vi "VMS_6_Master.vi"   [LabVIEW 2018]
uses:
  Common_FPGA_Timestamp/DataTypes/TimestampSettings.ctl
  <vilib>/rvi/Emulation/niFpgaGetClockAttributes.vi
  <vilib>/rvi/Emulation/niFpgaSctlEmulationGetInTimedLoop.vi
  <vilib>/rvi/Emulation/niFpgaEmulationReportErrorSimple.vi
  <vilib>/rvi/Emulation/niFpgaEmulationIsFPGAContextNoSignature.vi
  <vilib>/rvi/errors/niFpgaSetErrorForExecOnDevCompSimple.vi
  <vilib>/rvi/eio/common/nirviEmuReportErrorAndStop.vi
  <vilib>/rvi/DataTransferAndStorage/Container/Common/niFpgaContainerGetUniqueNameForEmu.vi
  <vilib>/rvi/FIFO/Fifo_Resource/nirvififoEmulationSetSize.vi
  <vilib>/rvi/FIFO/Fifo_Resource/nirviFifoEmulationQueueMgr.vi
  <instcachedir>/0/nirviFifoEmulationQueueMgr_E5CAEC123FF24DC58D834DCA3CDAA9B5.lvgen/nirviFifoEmulationQueueMgr_E5CAEC123FF24DC58D834DCA3CDAA9B5_022.vi
  <vilib>/Utility/error.llb/Clear Errors.vi
  <vilib>/rvi/FIFO/Fifo_Resource/nirvififoEmulationCreateLock.vi
  <vilib>/rvi/Emulation/niFpgaProcessEmulError.vi
  <vilib>/rvi/FIFO/Fifo_Resource/nirvififoEmulationObtainLock.vi
  <vilib>/rvi/FIFO/Fifo_Resource/nirvififoEmulationReleaseLock.vi
  <vilib>/rvi/occurrence/nirviWaitOnOccurrenceBase.vi
  <vilib>/rvi/errors/nirviReportUnexpectedCaseInternalError.vi
  <vilib>/rvi/errors/nirviReportUnexpectedCaseInternalError (U32).vi
  <vilib>/rvi/Emulation/niFpgaCriticalErrorInLSC.vi
  <vilib>/rvi/eio/common/nirviEmuTemplateMethod_errors.vi
  <vilib>/rvi/DataTransferAndStorage/Container/XNode/niFpgaContainer.xnode
  <vilib>/rvi/FIFO/Fifo_Resource/nirvififoEmulationRead.vi
  <vilib>/eio/EIONode/EIONode.xnode
  Common_FPGA_Timestamp/FPGATimestamp.lvlib
types:
  T1 = typedef "FPGATimestamp.lvlib/TimestampSettings.ctl" = cluster{"TimeSource":refnum<k21>, "TimeRegister":refnum<k21>, "IterationsPerMicrosecond":i16, "UpdateFIFO":refnum<k21>, "HealthAndStatusFIFO":refnum<k21>, "HealthAndStatusAddress":i16, "IterationsPerHealthAndStatusUpdate":i16}
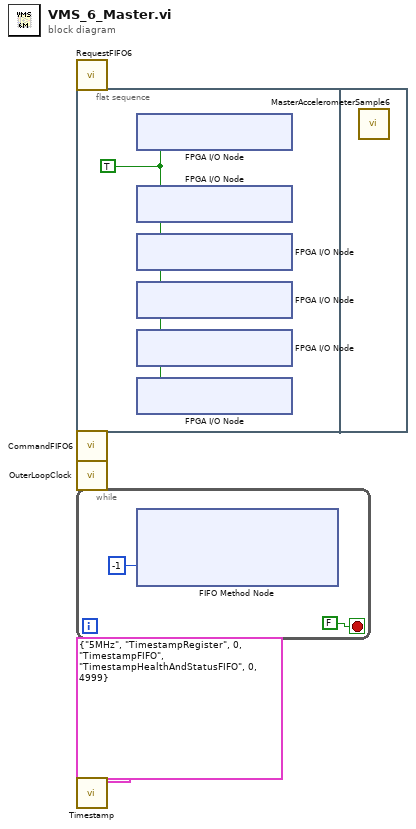
[diagram p0: block diagram]
diagram:
  n1 = call "RequestFIFO6.vi"() -> ()  [unwired: 12 in]
  n2 = flat-sequence {
    frame #0 {
      w2 = TRUE
      n3 = xnode "FPGA I/O Node"("Accelerometer1/Start"=w2) -> ()  [unwired: 1 in, 1 out]
      n4 = xnode "FPGA I/O Node"("Accelerometer2/Start"=w2) -> ()  [unwired: 1 in, 1 out]
      n5 = xnode "FPGA I/O Node"("Accelerometer3/Start"=w2) -> ()  [unwired: 1 in, 1 out]
      n6 = xnode "FPGA I/O Node"("Accelerometer4/Start"=w2) -> ()  [unwired: 1 in, 1 out]
      n7 = xnode "FPGA I/O Node"("Accelerometer5/Start"=w2) -> ()  [unwired: 1 in, 1 out]
      n8 = xnode "FPGA I/O Node"("Accelerometer6/Start"=w2) -> ()  [unwired: 1 in, 1 out]
    }
    frame #1 {
      n9 = call "MasterAccelerometerSample6.vi"() -> ()  [unwired: 12 in]
    }
  }
  n10 = call "CommandFIFO6.vi"() -> ()  [unwired: 12 in]
  n11 = call "OuterLoopClock.vi"() -> ()  [unwired: 12 in]
  n12 = while {
    stop <- FALSE stop-if-true
    n13 = xnode ("FIFO Method Node")("Timeout"=-1) -> ()  [unwired: 1 in, 3 out]
  }
  n14 = call "Timestamp.vi"("TimestampSettings"=T1 {"TimeSource"="5MHz", "TimeRegister"="TimestampRegister", "IterationsPerMicrosecond"=0, "UpdateFIFO"="TimestampFIFO", "HealthAndStatusFIFO"="TimestampHealthAndStatusFIFO", "HealthAndStatusAddress"=0, "IterationsPerHealthAndStatusUpdate"=4999}) -> ()  [unwired: 11 in]
